vi "Get Correct Target.vi"(1 "4":bool, 2 "2":bool, 3 "3":bool, 4 "Target Info":T2(array[cluster]), 5 "Target Found?":bool, 6 "1":bool) -> (0 "Selected Target Info":T1)   [LabVIEW 2011]
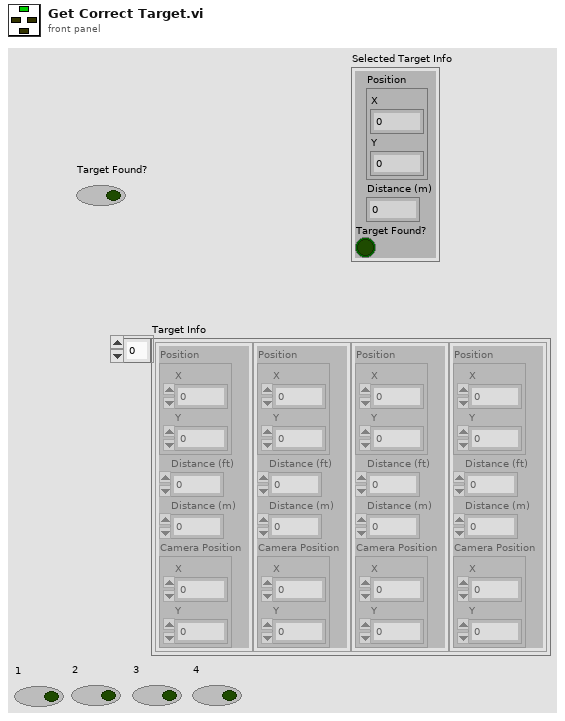
[diagram p1: front panel]
types:
  T1 = cluster{"Position":cluster{"X":dbl, "Y":dbl}, "Distance (m)":dbl, "Target Found?":bool}
  T2 = cluster{"Position":cluster{"X":dbl, "Y":dbl}, "Distance (ft)":dbl, "Distance (m)":dbl, "Camera Position":cluster{"X":dbl, "Y":dbl}}[]
  T3 = cluster{"Position":cluster{"X":dbl, "Y":dbl}, "Distance (ft)":dbl, "Distance (m)":dbl, "Camera Position":cluster{"X":dbl, "Y":dbl}}
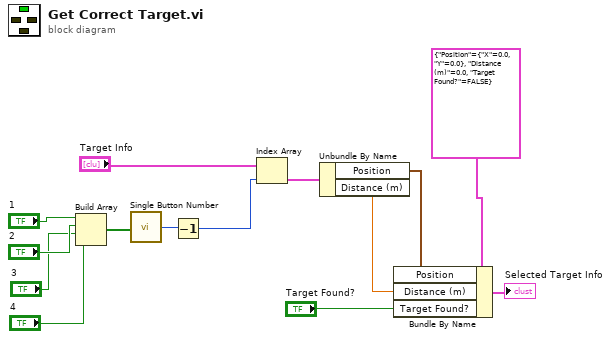
[diagram p0: block diagram]
diagram:
  n1 = Build Array("1", "2", "3", "4") -> (w10:bool[])
  n2 = call "Single Button Number.vi"("Bool Array"=w10) -> ("Number"=w9:i32)
  n3 = Decrement(x=w9) -> (x-1=w8:i32)
  n4 = Index Array(array="Target Info", index=w8) -> (element=w7:T3)
  n5 = Unbundle By Name(w7) -> ("Position"=w6:cluster{"X":dbl, "Y":dbl}, "Distance (m)"=w5:dbl)
  n6 = Bundle By Name(cluster=T1 {"Position"={"X"=0.0, "Y"=0.0}, "Distance (m)"=0.0, "Target Found?"=FALSE} ("input cluster"), "Position"=w6, "Distance (m)"=w5, "Target Found?"="Target Found?") -> (→"Selected Target Info":T1)
